vi "Set_K2400_Output_Off.vi"(8 "error in (no error)":errorcluster) -> (0 "error out":errorcluster)   [LabVIEW 2020]
uses:
  <instrlib>/Keithley 24XX/Keithley 24XX.lvlib
panel:
  out "VISA resource name out":refnum<visa-resource-name>
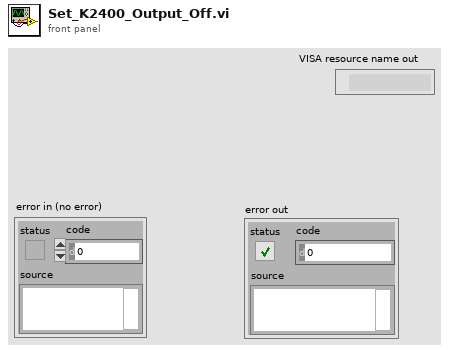
[diagram p1: front panel]
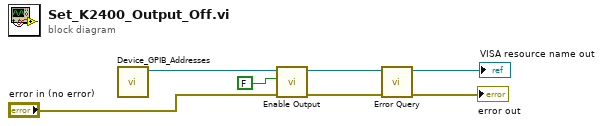
[diagram p0: block diagram]
diagram:
  n1 = call "Device_GPIB_Addresses.vi"() -> ("Keithley 2400 Address"=w1:refnum<visa-resource-name>)  [unwired: 9 in, 2 out]
  n2 = call <instrlib>:"Enable Output.vi"("error in (no error)"="error in (no error)", "Enable Output (T: Enable)"=FALSE, "VISA resource name"=w1) -> ("error out"=w5:errorcluster, "VISA resource name out"=w4:refnum<visa-resource-name>)  [unwired: 7 in]
  n3 = call <instrlib>:"Error Query.vi"("error in (no error)"=w5, "VISA resource name"=w4) -> ("error out"=→"error out":errorcluster, "VISA resource name out"=→"VISA resource name out":refnum<visa-resource-name>)  [unwired: 6 in, 2 out]
